vi "set_DC_Voltage.vi"(6 "error in (no error)":errorcluster, 8 "NoiseFrequency/Hz":i32[](array[numeric]) min=6 max=511, 9 "Use Noise Rejecting":bool, 10 "Messdauer/ms":i32, 11 "Einstellungen":T2={"Channel Name"="1", "Source Delay (Sec)"=0.5, "Measurement:Sense"=1008, "voltage level"=0.0, "voltage level range"=20.0, "current limit"=0.02, "current limit range"=0.02, "resource name"="PSU"} {"current limit range" format="%_6p"; "current limit" format="%_6p"; "voltage level range" format="%_6p"; "voltage level" format="%_6p"; "Measurement:Sense" items=["Local"=1008, "Remote"=1009]; "Source Delay (Sec)" format="%_6p"}) -> (0 "error out":errorcluster {"code" format="%.0x"}, 1 "Supply Output":T1 {"Current mean" format="%.8f"; "Voltage mean" format="%.8f"; "Voltage min" format="%#_8g"; "Voltage max" format="%#_8g"; "Current min" format="%#_8g"; "Current max" format="%#_8g"}, 2 "Current":waveform(dbl)(graph), 3 "Voltage":waveform(dbl)(graph))   [LabVIEW 2018]
doc: "Das VI configuriert die Power Supply und misst die beiden Kanäle zurück.\n\nBei Messzeit==0 erfolgt keine Messung.\nAb einer Meszeit von 1 ms wird zumindest eine Messung durchgeführt.\n\nDie Samplerate ist von der Noise Rejection abhängig,\nbei Noise Frequency = 50Hz -->Teiler = 60 beträgt diese 50 Samples/Sekunde\nbei Noise Frequency = 60Hz -->Teiler = 50 beträgt diese 60 Samples/Sekunde\nbei Noise Frequency = 50+60Hz -->Teiler = 300 beträgt diese 10 Samples / Sekunde"
uses:
  Type/SupplyConfig.ctl
  Type/SupplyOutput.ctl
  <instrlib>/niDCPower/nidcpower.llb/niDCPower Wait For Event - Event.ctl
panel:
  # "Einstellungen"
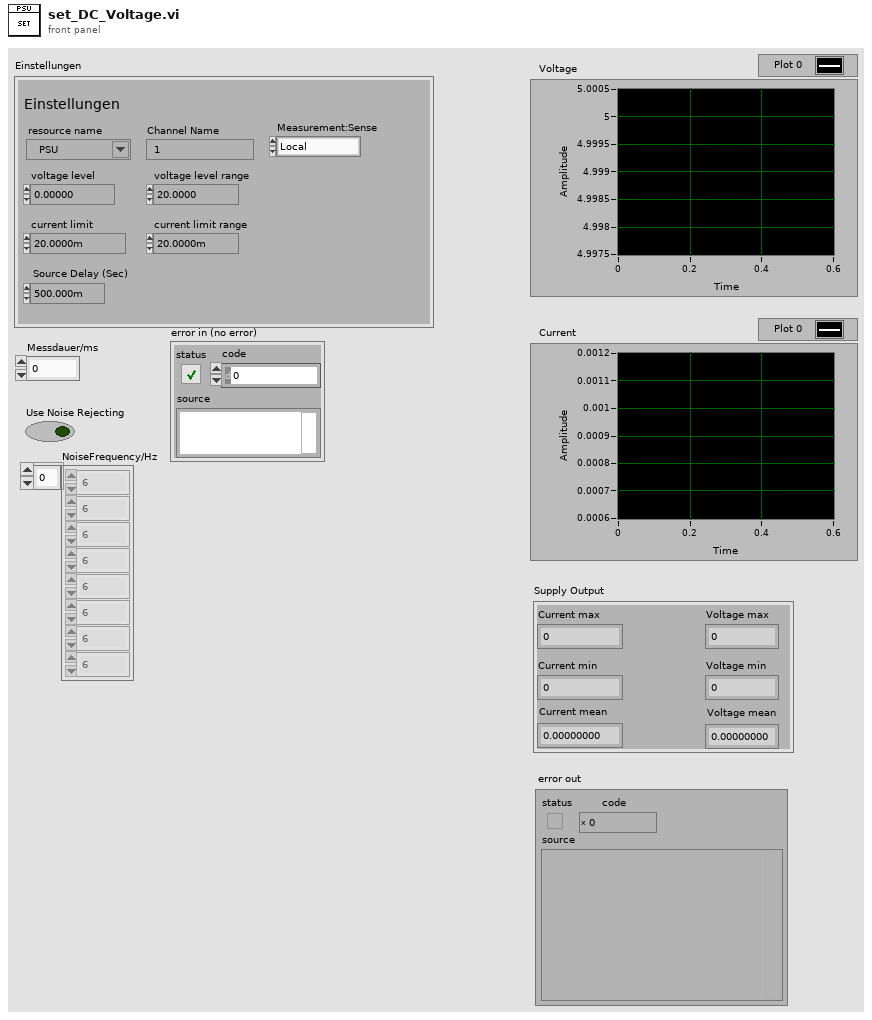
[diagram p1: front panel]
types:
  T1 = typedef "SupplyOutput.ctl" = cluster{"Current max":dbl, "Current min":dbl, "Voltage max":dbl, "Voltage min":dbl, "Voltage mean":dbl, "Current mean":dbl}
  T2 = typedef "SupplyConfig.ctl" = cluster{"Channel Name":string, "Source Delay (Sec)":dbl, "Measurement:Sense":i32, "voltage level":dbl, "voltage level range":dbl, "current limit":dbl, "current limit range":dbl, "resource name":refnum<k15>}
  T3 = typedef "niDCPower Wait For Event - Event.ctl" = i32
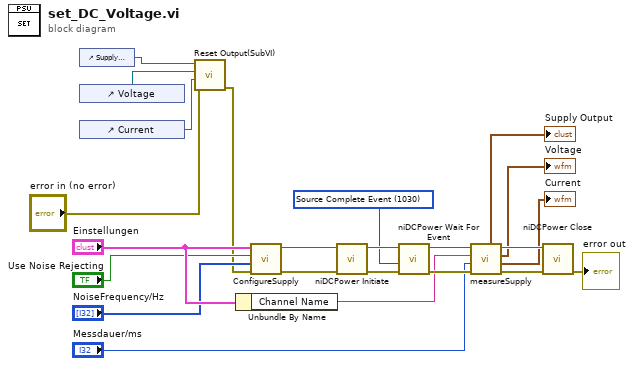
[diagram p0: block diagram]
diagram:
  w21 = T3 1030 items=["Source Complete Event"=1030, "Measure Complete Event"=1031, "Sequence Iteration Complete Event"=1032, "Sequence Engine Done Event"=1033, "Pulse Complete Event"=1051, "Ready For Pulse Trigger Event"=1052] ("event")
  n1 = control-ref of="Supply Output"() -> (w6:refnum<vi>)
  n2 = control-ref of="Voltage"() -> (w5:refnum<vi>)
  n3 = control-ref of="Current"() -> (w4:refnum<vi>)
  n4 = call "Reset Output(SubVI).vi"("error in (no error)"="error in (no error)", "WFGraph Refnum 2"=w4, "WFGraph Refnum"=w5, "Cluster in"=w6) -> ("error out"=w7:errorcluster)  [unwired: 7 in]
  n5 = Unbundle By Name("Einstellungen") -> ("Channel Name"=w13:string)
  n6 = call "ConfigureSupply.vi"("error in (no error)"=w7, "NoiseFrequency/Hz"="NoiseFrequency/Hz", "Use Noise Rejecting"="Use Noise Rejecting", "Einstellungen"="Einstellungen") -> ("error out"=w19:errorcluster, "instrument handle out"=w20:refnum<k15>)  [unwired: 6 in]
  n7 = call <instrlib>:"niDCPower Initiate.vi"("error in (no error)"=w19, "instrument handle"=w20) -> ("error out"=w22:errorcluster, "instrument handle out"=w23:refnum<k15>)  [unwired: 8 in]
  n8 = call <instrlib>:"niDCPower Wait For Event.vi"("error in (no error)"=w22, "event"=w21, "instrument handle"=w23) -> ("error out"=w17:errorcluster, "instrument handle out"=w18:refnum<k15>)  [unwired: 7 in]
  n9 = call "measureSupply.vi"("Supply instrument handle"=w18, "Supply Channel"=w13, "Messdauer/ms"="Messdauer/ms", "error in (no error)"=w17) -> ("Supply Output"=→"Supply Output":T1, "Supply instrument handle"=w15:refnum<k15>, "Supply Voltage"=→"Voltage":waveform(dbl), "Supply Current"=→"Current":waveform(dbl), "error out"=w16:errorcluster)  [unwired: 2 in]
  n10 = call <instrlib>:"niDCPower Close.vi"("error in (no error)"=w16, "instrument handle"=w15) -> ("error out"=→"error out":errorcluster)  [unwired: 9 in]
